vi "Demo_DecompressImageToMemory.vi"() -> ()   [LabVIEW 2024]
doc: "Decompress into memory an image in any formats\nsupported by QuickTime. You can speed up the operation by providing the source image format or use '****' to tell the VI to guess the format. \n\n© Ch. Salzmann, 1994-2003"
uses:
  <userlib>/ImageProcessing/QTLIB_2595_LV86/QT_Private.ctl
  <userlib>/ImageProcessing/QTLIB_2595_LV86/QT_Image.ctl
  <userlib>/ImageProcessing/QTLIB_2595_LV86/QT_Compression.ctl
panel:
  in  "Format":u16(ring)=10 items=["BMP", "JPEG", "MacPaint", "Photoshop", "PNG", "PICT", "QuickTime", "SG", "Targa", "TIFF", "Guess format"]
  in  "Compressed data":u8[](array[numeric])=[255, 216, 255, 224, 0, 16, 74, 70, 73, 70, 0, 1, 1, 1, 0, 72, 0, 72, 0, 0, 255, 254, 0, 12, 65, 112, 112, 108, 101, 77, 97, 114, 107, 10, 255, 219, 0, 132, 0, 7, 5, 6, 6, 6, 5, 7, 6, 6, 6, 8, 8, 7, 9, 11, 18, 12, 11, 10, 10, 11, 21, 15, 16, 13, 18, 25, 22, 27, 26, 25, 22, 24, 24, 28, 31, 40, 34, 28, 30, 38, 30, 24, 24, 35, 47, 35, 38, 41, 42, 45, 45, 45, 27, 33, 49, 52, 48, 43, 52, 40, 44, 45, 43, 1, 8, 8, 8, 11, 9, 11, 21, 12, 12, 21, 43, 29, 24, 29, 43, 43, 43, 43, 43, 43, 43, 43, 43, 43, 43, 43, 43, 43, 43, 43, 43, 43, 43, 43, 43, 43, 43, 43, 43, 43, 43, 43, 43, 43, 43, 43, 43, 43, 43, 43, 43, 43, 43, 43, 43, 43, 43, 43, 43, 43, 43, 43, 43, 43, 255, 196, 1, 162, 0, 0, 1, 5, 1, 1, 1, 1, 1, 1, 0, 0, 0, 0, 0, 0, 0, 0, 1, 2, 3, 4, 5, 6, 7, 8, 9, 10, 11, 1, 0, 3, 1, 1, 1, 1, 1, 1, 1, 1, 1, 0, 0, 0, 0, 0, 0, 1, 2, 3, 4, 5, 6, 7, 8, 9, 10, 11, 16, 0, 2, 1, 3, 3, 2, 4, 3, 5, 5, 4, 4, 0, 0, 1, 125, 1, 2, 3, 0, 4, 17, 5, 18, 33, 49, 65, 6, 19, 81, 97, 7, 34, 113, 20, 50, 129, 145, 161, 8, 35, 66, 177, 193, 21, 82, 209, 240, 36, 51, 98, 114, 130, 9, 10, 22, 23, 24, 25, 26, 37, 38, 39, 40, 41, 42, 52, 53, 54, 55, 56, 57, 58, 67, 68, 69, 70, 71, 72, 73, 74, 83, 84, 85, 86, 87, 88, 89, 90, 99, 100, 101, 102, 103, 104, 105, 106, 115, 116, 117, 118, 119, 120, 121, 122, 131, 132, 133, 134, 135, 136, 137, 138, 146, 147, 148, 149, 150, 151, 152, 153, 154, 162, 163, 164, 165, 166, 167, 168, 169, 170, 178, 179, 180, 181, 182, 183, 184, 185, 186, 194, 195, 196, 197, 198, 199, 200, 201, 202, 210, 211, 212, 213, 214, 215, 216, 217, 218, 225, 226, 227, 228, 229, 230, 231, 232, 233, 234, 241, 242, 243, 244, 245, 246, 247, 248, 249, 250, 17, 0, 2, 1, 2, 4, 4, 3, 4, 7, 5, 4, 4, 0, 1, 2, 119, 0, 1, 2, 3, 17, 4, 5, 33, 49, 6, 18, 65, 81, 7, 97, 113, 19, 34, 50, 129, 8, 20, 66, 145, 161, 177, 193, 9, 35, 51, 82, 240, 21, 98, 114, 209, 10, 22, 36, 52, 225, 37, 241, 23, 24, 25, 26, 38, 39, 40, 41, 42, 53, 54, 55, 56, 57, 58, 67, 68, 69, 70, 71, 72, 73, 74, 83, 84, 85, 86, 87, 88, 89, 90, 99, 100, 101, 102, 103, 104, 105, 106, 115, 116, 117, 118, 119, 120, 121, 122, 130, 131, 132, 133, 134, 135, 136, 137, 138, 146, 147, 148, 149, 150, 151, 152, 153, 154, 162, 163, 164, 165, 166, 167, 168, 169, 170, 178, 179, 180, 181, 182, 183, 184, 185, 186, 194, 195, 196, 197, 198, 199, 200, 201, 202, 210, 211, 212, 213, 214, 215, 216, 217, 218, 226, 227, 228, 229, 230, 231, 232, 233, 234, 242, 243, 244, 245, 246, 247, 248, 249, 250, 255, 192, 0, 17, 8, 0, 100, 0, 100, 3, 1, 34, 0, 2, 17, 1, 3, 17, 1, 255, 218, 0, 12, 3, 1, 0, 2, 17, 3, 17, 0, 63, 0, 244, 154, 40, 170, 55, 186, 148, 22, 119, 218, 117, 148, 169, 49, 150, 254, 71, 142, 34, 145, 146, 138, 86, 54, 115, 185, 186, 14, 20, 224, 117, 61, 134, 1, 35, 128, 230, 47, 81, 89, 75, 172, 39, 246, 148, 118, 82, 216, 222, 66, 147, 72, 208, 193, 115, 42, 42, 199, 52, 138, 172, 197, 84, 110, 222, 56, 71, 33, 153, 66, 144, 185, 4, 229, 114, 249, 245, 139, 40, 174, 244, 251, 80, 207, 51, 95, 79, 44, 17, 188, 75, 186, 53, 120, 213, 217, 195, 55, 69, 35, 99, 12, 117, 200, 60, 112, 216, 118, 11, 26, 84, 85, 27, 125, 74, 9, 245, 91, 221, 45, 18, 97, 61, 164, 113, 73, 35, 60, 101, 80, 137, 55, 237, 218, 79, 222, 251, 135, 36, 113, 219, 57, 4, 10, 58, 166, 190, 182, 50, 66, 176, 105, 151, 154, 130, 77, 39, 146, 146, 89, 188, 12, 12, 187, 153, 90, 60, 52, 138, 197, 151, 107, 22, 192, 194, 128, 196, 145, 181, 176, 88, 44, 110, 81, 88, 246, 250, 245, 188, 215, 233, 106, 45, 174, 86, 25, 103, 146, 218, 27, 166, 9, 229, 75, 52, 123, 183, 160, 1, 183, 130, 60, 185, 57, 101, 10, 118, 28, 19, 149, 204, 218, 150, 177, 167, 233, 250, 101, 198, 163, 44, 232, 240, 194, 178, 157, 177, 186, 150, 118, 137, 89, 157, 23, 158, 88, 8, 223, 140, 241, 180, 231, 24, 52, 89, 133, 141, 42, 43, 3, 74, 241, 61, 142, 163, 97, 115, 168, 8, 222, 27, 72, 24, 39, 153, 231, 65, 56, 119, 63, 192, 190, 68, 146, 101, 178, 84, 5, 234, 75, 40, 0, 147, 90, 154, 93, 236, 90, 158, 153, 103, 168, 192, 174, 176, 221, 64, 147, 162, 184, 1, 130, 186, 134, 0, 224, 158, 112, 125, 104, 105, 160, 177, 110, 138, 40, 164, 1, 69, 20, 80, 1, 84, 111, 236, 126, 215, 117, 166, 92, 121, 187, 62, 197, 114, 103, 219, 183, 59, 243, 12, 145, 227, 175, 31, 235, 51, 158, 122, 99, 190, 106, 245, 20, 1, 135, 109, 166, 106, 177, 235, 211, 106, 119, 58, 149, 156, 240, 62, 82, 56, 190, 198, 203, 36, 49, 118, 68, 127, 52, 129, 150, 1, 152, 236, 203, 16, 58, 0, 161, 109, 92, 233, 242, 221, 92, 105, 179, 205, 112, 155, 172, 174, 222, 224, 4, 140, 128, 234, 99, 150, 53, 94, 88, 224, 129, 32, 201, 238, 84, 240, 51, 198, 149, 20, 238, 23, 40, 197, 99, 229, 235, 55, 122, 159, 155, 159, 180, 91, 67, 7, 151, 183, 238, 249, 109, 43, 103, 57, 231, 62, 111, 76, 113, 183, 223, 140, 173, 115, 195, 243, 235, 18, 68, 211, 221, 217, 252, 155, 213, 93, 172, 67, 75, 110, 11, 18, 30, 222, 77, 217, 138, 93, 187, 114, 231, 112, 220, 138, 193, 87, 4, 30, 142, 138, 46, 199, 115, 156, 180, 240, 223, 217, 245, 230, 213, 126, 211, 9, 253, 228, 146, 239, 91, 125, 183, 50, 111, 207, 238, 229, 155, 119, 207, 18, 238, 249, 83, 104, 198, 200, 185, 59, 57, 216, 150, 43, 217, 33, 242, 197, 226, 68, 204, 207, 186, 72, 225, 249, 130, 16, 219, 118, 238, 36, 6, 92, 161, 201, 12, 14, 211, 242, 140, 241, 110, 138, 47, 113, 92, 231, 63, 225, 27, 23, 183, 47, 123, 173, 221, 125, 162, 240, 249, 98, 55, 178, 243, 108, 132, 98, 49, 40, 82, 54, 200, 91, 119, 239, 229, 4, 238, 193, 4, 12, 12, 100, 232, 248, 127, 76, 93, 23, 67, 176, 210, 146, 103, 152, 90, 192, 177, 121, 142, 73, 46, 64, 228, 242, 78, 6, 122, 46, 112, 6, 0, 224, 10, 210, 162, 139, 182, 59, 133, 20, 81, 72, 65, 69, 20, 80, 1, 69, 20, 80, 1, 69, 21, 204, 234, 183, 55, 186, 213, 253, 223, 135, 180, 169, 238, 108, 99, 129, 87, 237, 218, 146, 71, 204, 101, 182, 183, 145, 17, 36, 126, 240, 163, 110, 46, 3, 4, 5, 120, 203, 13, 173, 43, 129, 163, 121, 173, 218, 193, 114, 246, 86, 209, 205, 127, 126, 152, 223, 107, 104, 3, 188, 121, 25, 27, 216, 144, 145, 228, 114, 55, 178, 238, 193, 219, 147, 197, 65, 230, 120, 158, 235, 253, 93, 182, 155, 166, 161, 249, 149, 231, 119, 187, 147, 29, 149, 163, 93, 138, 173, 207, 36, 72, 192, 17, 129, 187, 59, 134, 173, 157, 172, 22, 86, 201, 109, 109, 30, 200, 147, 56, 4, 150, 36, 147, 146, 196, 158, 89, 137, 36, 146, 73, 36, 146, 73, 36, 212, 244, 92, 102, 31, 145, 226, 164, 249, 255, 0, 180, 244, 121, 246, 243, 229, 125, 130, 88, 183, 255, 0, 179, 191, 206, 109, 185, 233, 187, 107, 99, 174, 15, 74, 63, 181, 181, 43, 79, 249, 10, 232, 115, 42, 117, 51, 233, 239, 246, 200, 212, 116, 0, 174, 213, 148, 182, 123, 44, 108, 0, 32, 231, 174, 221, 202, 40, 184, 92, 130, 206, 238, 214, 250, 217, 46, 172, 174, 97, 185, 183, 124, 236, 150, 23, 14, 141, 131, 131, 130, 56, 60, 130, 63, 10, 158, 176, 53, 141, 50, 246, 43, 191, 237, 189, 18, 103, 75, 200, 213, 140, 246, 89, 253, 206, 160, 54, 224, 43, 2, 64, 73, 62, 85, 2, 94, 160, 12, 16, 202, 48, 52, 116, 109, 74, 13, 95, 77, 135, 80, 182, 73, 163, 73, 55, 3, 28, 241, 152, 228, 141, 149, 138, 178, 50, 158, 140, 172, 8, 62, 227, 189, 22, 234, 5, 234, 40, 162, 144, 130, 138, 40, 160, 2, 138, 40, 160, 12, 221, 122, 246, 93, 63, 75, 150, 123, 117, 70, 185, 102, 72, 32, 18, 2, 83, 205, 145, 214, 56, 203, 224, 231, 110, 231, 93, 216, 231, 25, 198, 77, 79, 166, 89, 69, 167, 88, 65, 101, 11, 59, 172, 75, 131, 36, 132, 23, 145, 186, 179, 185, 0, 101, 152, 146, 204, 123, 146, 79, 122, 206, 213, 63, 127, 226, 61, 6, 211, 238, 249, 63, 104, 190, 221, 215, 59, 16, 67, 179, 30, 255, 0, 105, 221, 159, 246, 49, 142, 114, 55, 41, 244, 24, 81, 69, 20, 132, 67, 12, 222, 108, 151, 9, 183, 30, 76, 129, 51, 158, 191, 42, 182, 127, 241, 239, 210, 166, 170, 54, 174, 145, 207, 168, 187, 176, 85, 19, 140, 150, 56, 31, 234, 163, 169, 252, 201, 100, 255, 0, 82, 155, 23, 251, 242, 2, 63, 37, 235, 249, 227, 241, 169, 82, 10, 48, 149, 72, 243, 61, 174, 245, 233, 191, 245, 166, 228, 196, 133, 25, 98, 0, 206, 57, 172, 75, 143, 248, 151, 120, 142, 218, 100, 255, 0, 81, 171, 102, 222, 68, 29, 167, 68, 103, 73, 49, 192, 230, 52, 145, 89, 142, 73, 217, 8, 28, 3, 90, 201, 2, 43, 7, 98, 210, 72, 58, 59, 242, 71, 211, 176, 252, 43, 39, 198, 63, 39, 135, 47, 46, 250, 253, 135, 101, 246, 223, 239, 253, 157, 214, 109, 153, 237, 187, 203, 219, 158, 113, 156, 224, 227, 21, 81, 191, 82, 228, 162, 157, 162, 239, 253, 127, 95, 228, 110, 81, 69, 20, 16, 20, 81, 69, 0, 20, 81, 69, 0, 97, 223, 254, 235, 197, 122, 45, 196, 156, 69, 37, 181, 213, 170, 183, 172, 172, 98, 145, 87, 241, 72, 37, 57, 233, 242, 227, 57, 32, 29, 202, 199, 241, 52, 50, 155, 8, 239, 173, 162, 121, 46, 116, 249, 210, 238, 53, 141, 75, 59, 42, 241, 42, 162, 255, 0, 19, 52, 77, 42, 40, 61, 216, 114, 14, 8, 212, 130, 104, 174, 33, 142, 120, 37, 73, 97, 145, 67, 164, 136, 193, 149, 212, 140, 130, 8, 234, 8, 239, 77, 236, 50, 74, 163, 168, 223, 125, 151, 203, 130, 8, 190, 209, 125, 62, 68, 22, 225, 182, 238, 198, 50, 204, 112, 118, 162, 228, 110, 108, 28, 100, 0, 11, 50, 169, 143, 80, 189, 149, 102, 93, 63, 79, 84, 147, 80, 145, 119, 124, 224, 152, 237, 208, 146, 60, 201, 48, 71, 25, 4, 42, 130, 11, 144, 64, 32, 6, 101, 147, 78, 211, 210, 203, 204, 145, 167, 154, 234, 234, 92, 121, 183, 51, 237, 243, 28, 12, 237, 95, 148, 5, 10, 50, 112, 20, 1, 146, 78, 50, 204, 72, 33, 108, 44, 140, 9, 190, 230, 81, 113, 118, 196, 188, 147, 108, 218, 11, 30, 62, 85, 231, 104, 3, 0, 12, 147, 128, 50, 88, 228, 155, 180, 81, 74, 214, 29, 216, 86, 31, 140, 254, 111, 10, 106, 214, 235, 204, 183, 86, 207, 107, 10, 255, 0, 122, 89, 71, 151, 26, 251, 101, 221, 70, 79, 3, 57, 36, 14, 107, 114, 176, 245, 143, 244, 237, 87, 76, 210, 147, 230, 72, 228, 23, 183, 99, 176, 72, 243, 229, 2, 71, 33, 140, 219, 25, 122, 6, 16, 201, 201, 193, 5, 173, 193, 27, 148, 81, 69, 33, 5, 20, 81, 64, 5, 20, 81, 64, 5, 114, 87, 51, 203, 225, 169, 174, 32, 187, 185, 75, 95, 13, 206, 161, 109, 46, 163, 83, 187, 78, 149, 136, 81, 27, 100, 50, 136, 201, 37, 149, 155, 10, 152, 216, 70, 221, 130, 186, 218, 142, 120, 98, 184, 134, 72, 39, 137, 37, 134, 69, 40, 241, 186, 134, 87, 82, 48, 65, 7, 168, 35, 181, 52, 198, 136, 52, 251, 40, 172, 97, 104, 227, 103, 146, 73, 27, 204, 154, 105, 8, 50, 76, 228, 0, 89, 136, 3, 156, 0, 48, 0, 0, 0, 0, 0, 0, 45, 214, 31, 246, 126, 165, 166, 255, 0, 200, 22, 120, 100, 181, 31, 119, 79, 187, 249, 99, 140, 118, 88, 165, 80, 90, 53, 25, 39, 12, 178, 12, 0, 170, 16, 10, 63, 183, 39, 183, 227, 83, 208, 181, 43, 96, 62, 83, 44, 17, 139, 184, 217, 189, 20, 68, 90, 77, 167, 146, 25, 145, 120, 28, 224, 144, 40, 181, 192, 220, 162, 176, 255, 0, 225, 36, 178, 111, 150, 27, 45, 98, 89, 79, 8, 159, 217, 87, 49, 238, 61, 134, 231, 69, 85, 207, 171, 16, 7, 114, 7, 52, 125, 175, 196, 55, 156, 90, 233, 112, 233, 168, 120, 50, 234, 18, 9, 100, 83, 215, 34, 24, 152, 171, 41, 224, 100, 202, 164, 28, 156, 112, 55, 22, 97, 98, 125, 115, 89, 131, 74, 142, 40, 177, 231, 234, 55, 91, 210, 202, 205, 73, 223, 115, 32, 82, 219, 70, 1, 218, 189, 50, 231, 229, 92, 228, 145, 70, 131, 99, 117, 107, 108, 103, 213, 37, 134, 125, 90, 227, 230, 185, 154, 37, 33, 58, 146, 177, 160, 39, 33, 16, 28, 14, 153, 229, 136, 220, 205, 151, 233, 250, 77, 189, 156, 205, 119, 35, 189, 222, 160, 203, 177, 239, 110, 21, 12, 204, 153, 7, 102, 85, 64, 85, 224, 124, 170, 0, 207, 36, 22, 36, 157, 42, 0, 40, 162, 138, 66, 10, 40, 162, 128, 10, 40, 162, 128, 10, 40, 162, 128, 10, 40, 162, 128, 10, 40, 162, 128, 10, 40, 162, 128, 10, 40, 162, 128, 10, 40, 162, 128, 63, 255, 217]
  out "The image":picture caption="new picture"
  out "error out":errorcluster={"status"=TRUE, "code"=0, "source"=""}
  # "Decompress into memory an image in any formats\nsupported by QuickTime\n© Ch. Salzmann, 1994-2005"
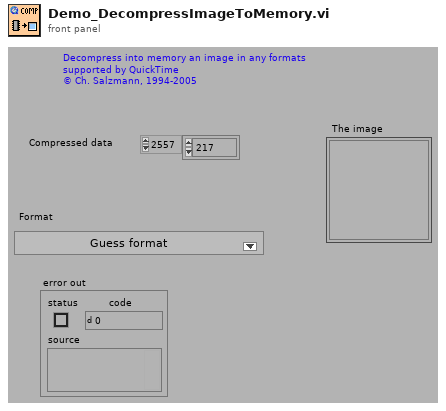
[diagram p1: front panel]
types:
  T1 = typedef "QT_Compression.ctl" = cluster{"Compression":i32, "Format":i32, "Codec":i32, "Comp. Quality":i32, "Key Frame":i32, "Dialogs":u32}
  T2 = typedef "QT_Image.ctl" = cluster{"Width":i32, "Height":i32, "Depth":i32, "data":u8[], "Compressed data":u8[], "Color table":u32[], "Duration":i32, "Options":i32, "Timestamp":i32, "ID":i32, "Reserved":i32, "Dialogs":u32}
  T3 = typedef "QT_Private.ctl" = cluster{"reserved 1":i32, "reserved 2":i32, "reserved 3":i32, "reserved 4":i32}
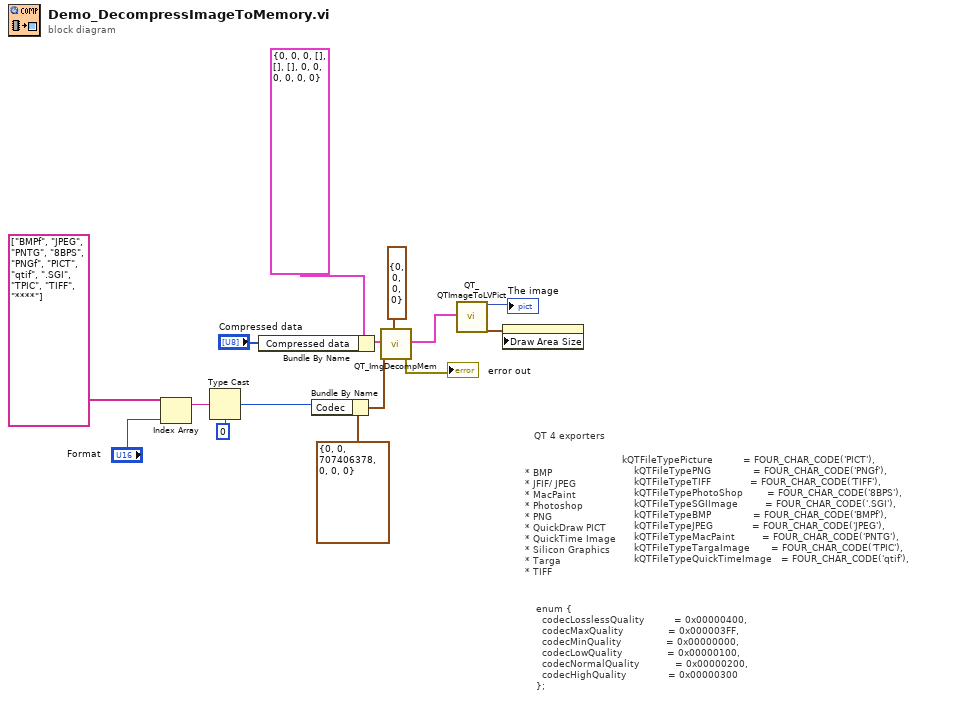
[diagram p0: block diagram]
diagram:
  # "QT 4 exporters"
  # "* BMP\n*\tJFIF/ JPEG \n*\tMacPaint\n*\tPhotoshop \n*\tPNG\n*\tQuickDraw PICT \n*\tQuickTime Image \n*\tSilicon Graphics\n*\tTarga\n*\tTIFF"
  # "kQTFileTypePicture          = FOUR_CHAR_CODE('PICT'),\n    kQTFileTypePNG              = FOUR_CHAR_CODE('PNGf'),\n    kQTFileTypeTIFF             = FOUR_CHAR_CODE('TIFF'),\n    kQTFileTypePhotoShop        = FOUR_CHAR_CODE('8BPS'),\n    kQTFileTypeSGIImage         = FOUR_CHAR_CODE('.SGI'),\n    kQTFileTypeBMP              = FOUR_CHAR_CODE('BMPf'),\n    kQTFileTypeJPEG             = FOUR_CHAR_CODE('JPEG'),\n    kQTFileTypeMacPaint         = FOUR_CHAR_CODE('PNTG'),\n    kQTFileTypeTargaImage       = FOUR_CHAR_CODE('TPIC'),\n    kQTFileTypeQuickTimeImage   = FOUR_CHAR_CODE('qtif'),"
  # "enum {\n  codecLosslessQuality          = 0x00000400,\n  codecMaxQuality               = 0x000003FF,\n  codecMinQuality               = 0x00000000,\n  codecLowQuality               = 0x00000100,\n  codecNormalQuality            = 0x00000200,\n  codecHighQuality              = 0x00000300\n};"
  n1 = Index Array(array=string[] ["BMPf", "JPEG", "PNTG", "8BPS", "PNGf", "PICT", "qtif", ".SGI", "TPIC", "TIFF", "****"], index="Format") -> (element=w5:string)
  n2 = Type Cast(type=0 ("Format"), x=w5) -> (*(type *) &x=w1:i32)
  n3 = Bundle By Name(cluster=T2 {"Width"=0, "Height"=0, "Depth"=0, "data"=[], "Compressed data"=[], "Color table"=[], "Duration"=0, "Options"=0, "Timestamp"=0, "ID"=0, "Reserved"=0, "Dialogs"=0} ("Image In"), "Compressed data"="Compressed data") -> (w9:T2)
  n4 = Bundle By Name(cluster=T1 {"Compression"=0, "Format"=0, "Codec"=707406378, "Comp. Quality"=0, "Key Frame"=0, "Dialogs"=0} ("Compression Settings"), "Codec"=w1) -> (w7:T1)
  n5 = call <userlib>:"QT_ImgDecompMem.vi"("Image In"=w9, "Compression Settings"=w7, "Private"=T3 {"reserved 1"=0, "reserved 2"=0, "reserved 3"=0, "reserved 4"=0}) -> ("Image/Movie Out"=w11:T2, "error out"=→"error out":errorcluster)  [unwired: 6 in, 9 out]
  n6 = call <userlib>:"QT_QTImageToLVPict.vi"("Image/Movie Out"=w11) -> ("Picture color"=→"The image":picture, "Pict Draw Area Size"=w13:cluster{"Width":i16, "Height":i16})  [unwired: 2 in, 15 out]
  n7 = property on="The image" class="Pict"("Draw Area Size"=w13) -> ()  [unwired: 2 in, 2 out]
